vi "FT10_Connect FPGA_7854R Handler.vi"(8 "error in":errorcluster, 10 "Message Data":variant, 11 "Message Handling Cluster in":T1) -> (0 "error out":errorcluster, 2 "PXI-7854R Connected?":bool, 3 "Message Handling Cluster out":T1)   [LabVIEW 2024]
uses:
  Controls/Control_Message Handling Cluster.ctl
  Controls/Control_M4X Connection.ctl
  Controls/Control_PXI-7854R FPGA Reference.ctl
  Controls/Control_PXI-7854R Connect Disconnect Cluster.ctl
  Controls/Control_PXI-7854R Resource.ctl
  Controls/Control_PXI-7854R 75kHz Bool.ctl
  Controls/Control_PXI-7854R uSec Off Numeric.ctl
  Controls/Control_PXI-7854R uSec On Numeric.ctl
  Controls/Control_PXI-7854R Connect Disconnect Bool.ctl
  <vilib>/FPGAPlugInAG/Dynamic/niLvFpga_Close_Dynamic.vi
  <vilib>/FPGAPlugInAG/PXI-7854R/niLvFpga_Open_PXI-7854R.vi
  <vilib>/rvi/interface/common/dynamic/niFpgaDynamicAddResources.vi
  <vilib>/Utility/error.llb/Error Cluster From Error Code.vi
  <vilib>/rvi/errors/niLvFpgaAdjustHostInterfaceError.vi
  <vilib>/rvi/interface/nirviCloseFPGA/nirviCloseFPGA.xnode
  <vilib>/rvi/interface/nirviOpenFPGA/nirviOpenFPGA.xnode
  FPGA Bitfiles/5_21_2024_FT10_FPGA_7854R_Main BitFile.lvbitx
  <vilib>/rvi/interface/nirviReadWriteControl/nirviReadWriteControl.xnode
  NiFpgaLv.dll
  <vilib>/rvi/interface/Simulation/niFpgaSimulationCallBeginRW.vi
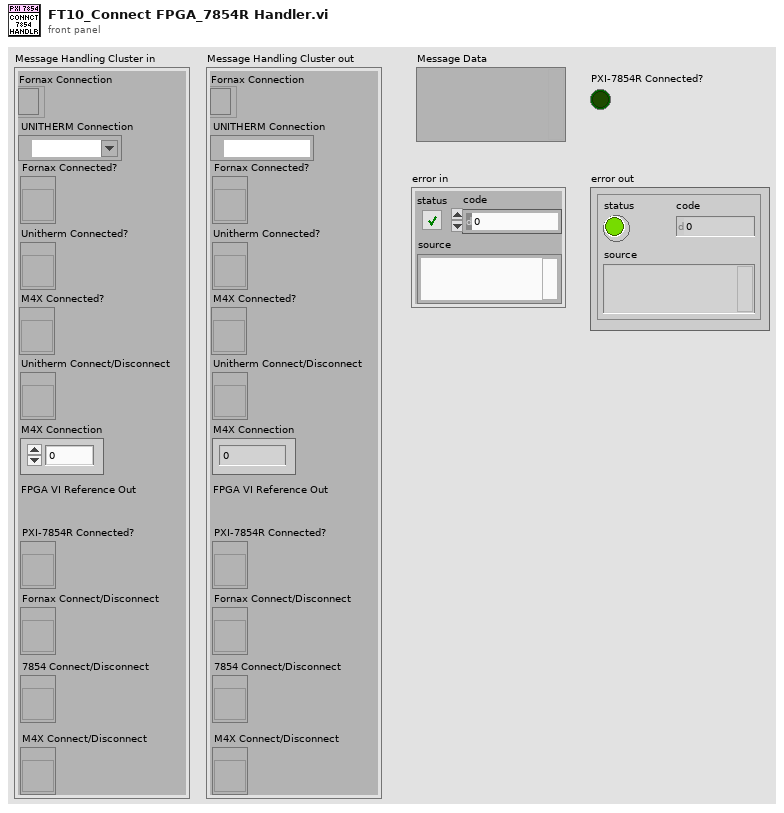
[diagram p1: front panel]
types:
  T1 = typedef "Control_Message Handling Cluster.ctl" = cluster{"Fornax Connected?":refnum<vi>, "Unitherm Connected?":refnum<vi>, "M4X Connected?":refnum<vi>, "Unitherm Connect/Disconnect":refnum<vi>, "Fornax Connection":refnum<k5>, "UNITHERM Connection":refnum<visa-resource-name>, "M4X Connection":T2, "PXI-7854R FPGA Reference":T3, "PXI-7854R Connected?":refnum<vi>, "Fornax Connect/Disconnect":refnum<vi>, "7854 Connect/Disconnect":refnum<vi>, "M4X Connect/Disconnect":refnum<vi>}
  T2 = typedef "Control_M4X Connection.ctl" = u32
  T3 = typedef "Control_PXI-7854R FPGA Reference.ctl" = refnum<k20>
  T4 = typedef "Control_PXI-7854R Connect Disconnect Cluster.ctl" = cluster{"PXI-7854R Resource":T5, "75kHz":T6, "uSec Off":T7, "uSec On":T8, "7854 Connect/Disconnect":T9}
  T5 = typedef "Control_PXI-7854R Resource.ctl" = tag
  T6 = typedef "Control_PXI-7854R 75kHz Bool.ctl" = bool
  T7 = typedef "Control_PXI-7854R uSec Off Numeric.ctl" = u16
  T8 = typedef "Control_PXI-7854R uSec On Numeric.ctl" = u16
  T9 = typedef "Control_PXI-7854R Connect Disconnect Bool.ctl" = bool
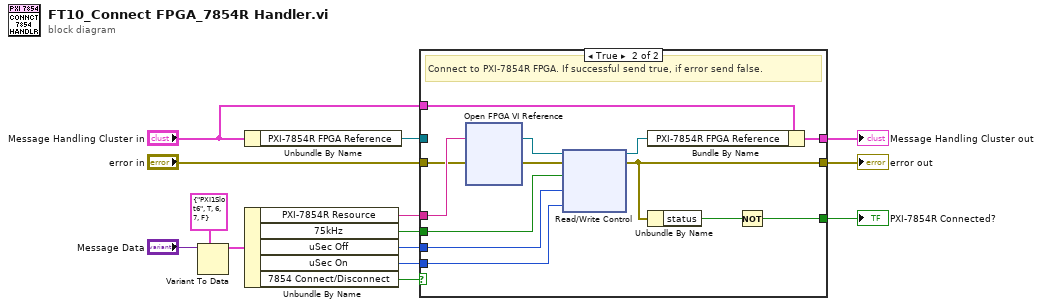
[diagram p0: block diagram]
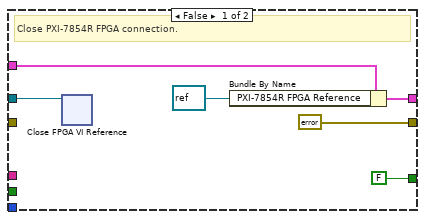
[diagram p2: hidden frame]
diagram:
  n1 = Variant To Data(type=T4 {"PXI-7854R Resource"="PXI1Slot6", "75kHz"=TRUE, "uSec Off"=6, "uSec On"=7, "7854 Connect/Disconnect"=FALSE}, Variant="Message Data") -> (data=w7:T4)  [unwired: 1 in, 1 out]
  n2 = Unbundle By Name("Message Handling Cluster in") -> ("PXI-7854R FPGA Reference"=w4:T3)
  n3 = Unbundle By Name(w7) -> ("PXI-7854R Resource"=w12:T5, "75kHz"=w8:T6, "uSec Off"=w9:T7, "uSec On"=w10:T8, "7854 Connect/Disconnect"=w11:T9)
  n4 = case shown="True" w11 {
    tunnel: w8 -> [_ w33]
    tunnel: w9 -> [_ w32]
    tunnel: w10 -> [_ w31]
    tunnel: w4 -> [w19 _]
    tunnel: [errorcluster {"status"=FALSE, "code"=0, "source"=""} ("error out") w23] -> w14
    tunnel: w12 -> [_ w29]
    tunnel: "error in" -> [_ w27]
    tunnel: "Message Handling Cluster in" -> [w18 w26]
    tunnel: [w17 w24] -> w2
    tunnel: [FALSE w21] -> w1
    frame False {
      # "Close PXI-7854R FPGA connection."
      n5 = xnode "Close FPGA VI Reference"("FPGA VI Reference In"=w19) -> ()  [unwired: 1 in, 1 out]
      n6 = Bundle By Name(cluster=w18, "PXI-7854R FPGA Reference"=refnum<k20> refnum ("FPGA VI Reference Out")) -> (w17:T1)
    }
    frame True {
      # "Connect to PXI-7854R FPGA. If successful send true, if error send false."
      n7 = xnode "Open FPGA VI Reference"("error in"=w27, "resource name"=w29) -> ("FPGA VI Reference Out"=w30:refnum<k20>, "error out"=w28:errorcluster)
      n8 = xnode "Read/Write Control"("FPGA VI Reference In"=w30, "error in"=w28, "75kHz"=w33, "uSec Off"=w32, "uSec On"=w31) -> ("FPGA VI Reference Out"=w25:refnum<k20>, "error out"=w23:errorcluster)
      n9 = Bundle By Name(cluster=w26, "PXI-7854R FPGA Reference"=w25) -> (w24:T1)
      n10 = Unbundle By Name(w23) -> ("status"=w22:bool)
      n11 = Not(x=w22) -> (.not. x?=w21:bool)
    }
  }
  "error out" <- w14
  "Message Handling Cluster out" <- w2
  "PXI-7854R Connected?" <- w1
